vi "AcqContinue.vi"(6 "Delay between send and receive [ms]":i32=100, 8 "error in (no error)":errorcluster, 11 "SCD in":refnum<class "SCD.lvclass">) -> (0 "error out":errorcluster, 3 "SCD out":refnum<class "SCD.lvclass">)   [LabVIEW 2020, in "horiba.lvlib" / "SCD.lvclass"]
doc: "Restart a paused acquisition.\nAn error will be returned if continue is received when not paused."
uses:
  SCD.lvclass
  SCD.lvclass/SCD.ctl
  GenericDevice/GenericDevice.lvclass
  ca73f763-8e2b-4d84-8e4e-0e6044455bd1.vi
panel:
  # "Connector Pane"
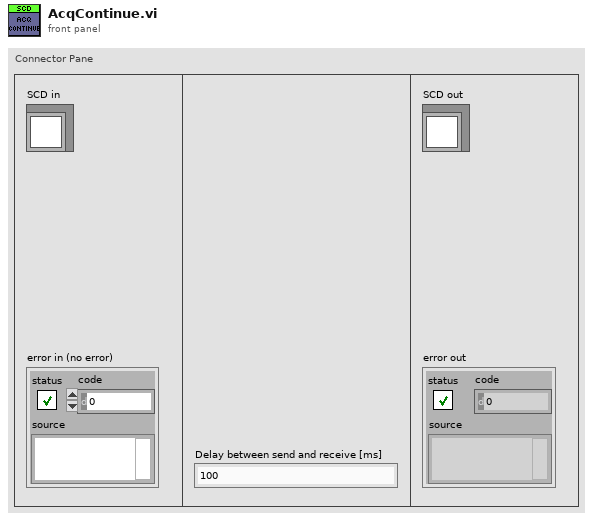
[diagram p1: front panel]
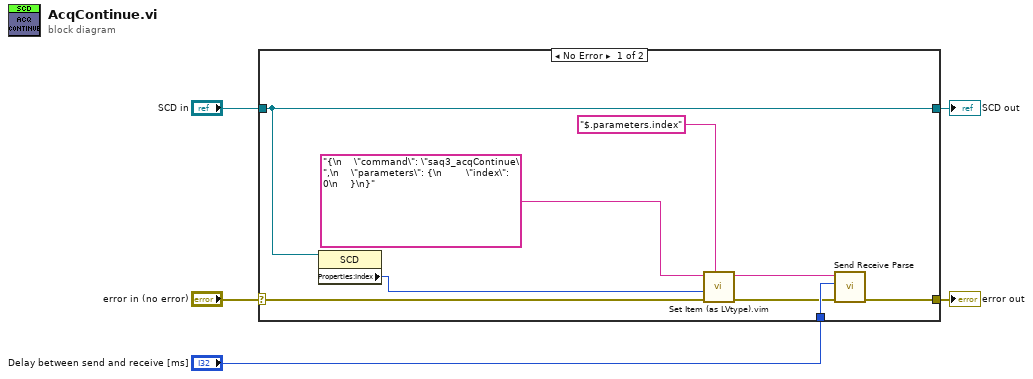
[diagram p0: block diagram]
diagram:
  n1 = case shown="No Error" "error in (no error)" {
    selector: "error in (no error)" -> [w13 w16]
    tunnel: [w12 w16] -> w1
    tunnel: [w14 w15] -> w3
    tunnel: "SCD in" -> [w14 w15]
    tunnel: "Delay between send and receive [ms]" -> [w11 _]
    frame No Error {
      n2 = property class="SCD"(reference=w14) -> ("Properties:Index"=w6:i32)  [unwired: 1 in, 2 out]
      n3 = call "Set Item (as LVtype).vim"("$Path or Item Name"="$.parameters.index", "error in (no error)"=w13, "Anything"=w6, "JSON"="{\n    \"command\": \"saq3_acqContinue\",\n    \"parameters\": {\n        \"index\": 0\n    }\n}") -> ("error out"=w10:errorcluster, "<JSON>"=w8:string)  [unwired: 4 in, 1 out]
      n4 = call "Send Receive Parse.vi"("error in"=w10, "Delay between send and receive [ms]"=w11, "<JSON>"=w8) -> ("error out"=w12:errorcluster)  [unwired: 6 in, 2 out]
    }
    frame Error {
    }
  }
  "error out" <- w1
  "SCD out" <- w3
